vi "UDP Connection Manager.vi"(7 "Action":T1, 8 "error in (no error)":errorcluster, 11 "UDP Port":u16) -> (0 "error out":errorcluster, 3 "connection ID out":refnum<k16>)   [LabVIEW 2021]
uses:
  Action.ctl
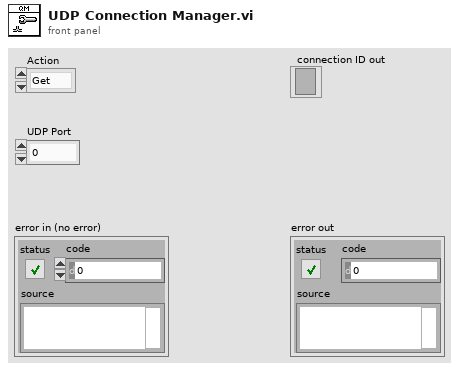
[diagram p1: front panel]
types:
  T1 = typedef "Action.ctl" = enum16{"Get", "Close"}
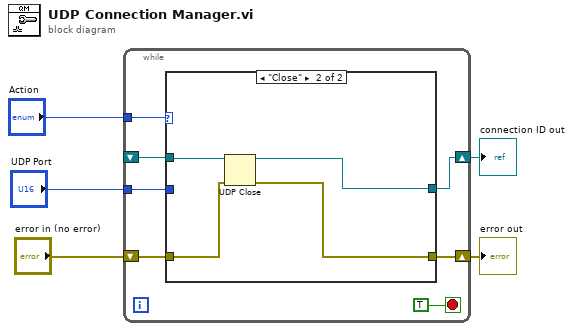
[diagram p0: block diagram]
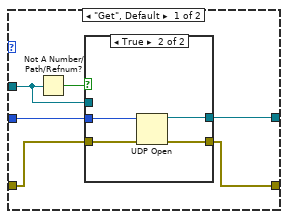
[diagram p2: hidden frame]
diagram:
  n1 = while {
    tunnel: "Action" -> [w12]
    tunnel: "UDP Port" -> [w11]
    shift-right: [w10] -> w2
    shift-left: _ -> [w9]
    shift-right: [w7] -> w1
    shift-left: "error in (no error)" -> [w8]
    stop <- TRUE stop-if-true
    n2 = case shown="\"Close\"" w12 {
      tunnel: w11 -> [w18 _]
      tunnel: [w17 w27] -> w10
      tunnel: w9 -> [w14 w28]
      tunnel: w8 -> [w15 w26]
      tunnel: [w13 w25] -> w7
      frame "Get", Default {
        n3 = Not A Number/Path/Refnum?(number/path/refnum=w14) -> (NaN/Path/Refnum?=w16:bool)
        n4 = case shown="True" w16 {
          tunnel: w18 -> [_ w24]
          tunnel: [w20 w23] -> w17
          tunnel: w15 -> [w19 w22]
          tunnel: [w19 w21] -> w13
          tunnel: w14 -> [w20 _]
          frame False {
          }
          frame True {
            n5 = UDP Open(8:w22, 11:w24) -> (port=w23:refnum<k16>, 0:w21:errorcluster)  [unwired: 3 in, 1 out]
          }
        }
      }
      frame "Close" {
        n6 = UDP Close(connection ID=w28, 8:w26) -> (connection ID out=w27:refnum<k16>, error out=w25:errorcluster)
      }
    }
  }
  "connection ID out" <- w2
  "error out" <- w1
